vi "judgetocarryon.vi"(6 "next_x":dbl, 7 "next_y":dbl, 9 "cur_y":dbl, 10 "cur_x":dbl, 11 "threshold":dbl) -> (3 "carryon":i32)   [LabVIEW 2015]
uses:
  <vilib>/imath/engines/lvmath2/RunTimeEngine/ArithmeticOperatorToken/NIMS_ArithmeticOperator_power(S).vi
  <instcachedir>/0/NIMS_ArithmeticOperator_power(S)_DFB67823F1414E5097C86E39787D8CA8.lvgen/NIMS_ArithmeticOperator_power(S)_DFB67823F1414E5097C86E39787D8CA8_014.vi
  <vilib>/imathl/engines/lvmath/Functions/Error Handling/Create Error.vi
  <vilib>/imath/engines/lvmath2/RunTimeEngine/NodeEndStatement/NIMS_NodeEndStatement_Output.vi
  <instcachedir>/0/NIMS_NodeEndStatement_Output_53EC0D466D134D7ABD903AC30B43404B.lvgen/NIMS_NodeEndStatement_Output_53EC0D466D134D7ABD903AC30B43404B_011.vi
  <vilib>/imath/engines/lvmath2/RunTimeEngine/ErrorHandling/NIMS_Finalize Error.vi
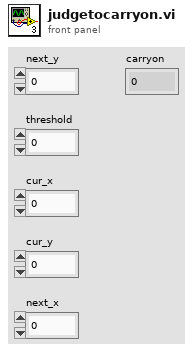
[diagram p1: front panel]
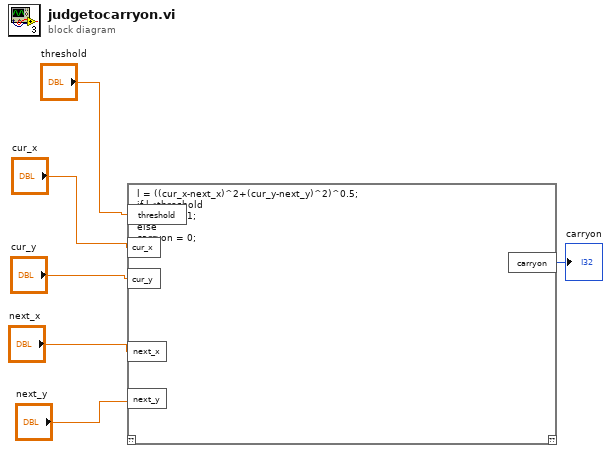
[diagram p0: block diagram]
diagram:
  n1 = mathscript code="l = ((cur_x-next_x)^2+(cur_y-next_y)^2)^0.5;\nif l<threshold\ncarryon = 1;\nelse\ncarryon = 0;\nend"("threshold"="threshold", "cur_x"="cur_x", "cur_y"="cur_y", "next_x"="next_x", "next_y"="next_y") -> ("carryon"=→"carryon":i32)  [unwired: 1 in, 1 out]
